vi "Update OccupancyGrid with Forget_factor.vi"(8 "error in (no error)":errorcluster, 11 "Probabilistic_OccupancyGrid in":refnum<class "Probabilistic_OccupancyGrid.lvclass">) -> (0 "error out":errorcluster, 3 "Probabilistic_OccupancyGrid out":refnum<class "Probabilistic_OccupancyGrid.lvclass">)   [LabVIEW 2017, in "Probabilistic_OccupancyGrid.lvclass"]
doc: "Update all cell costs with forget factor f\nlog(odd(ci,j.=occupied))= log(odd(ci,j.=occupied))+f *sign(log(odd(ci,j.=occupied)))\nCells not updated recently would have costs linearly reduced to 0"
uses:
  Probabilistic_OccupancyGrid.lvclass
  Probabilistic_OccupancyGrid.lvclass/Probabilistic_OccupancyGrid.ctl
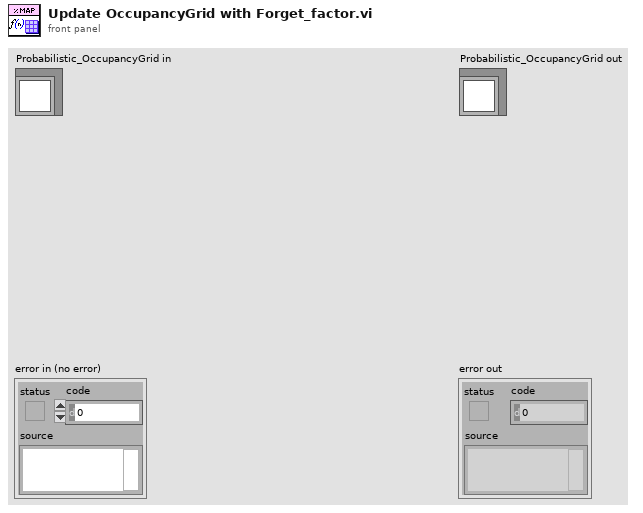
[diagram p1: front panel]
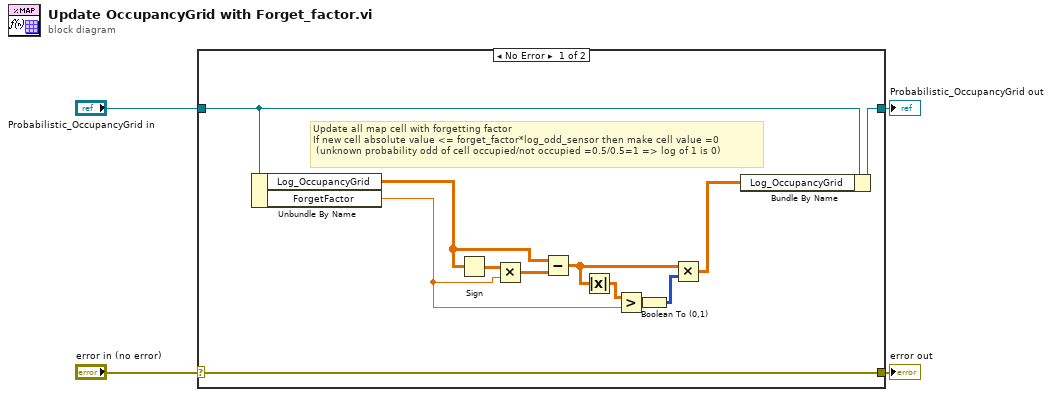
[diagram p0: block diagram]
diagram:
  n1 = case shown="No Error" "error in (no error)" {
    selector: "error in (no error)" -> [w16 w18]
    tunnel: [w16 w18] -> w3
    tunnel: [w8 w17] -> w1
    tunnel: "Probabilistic_OccupancyGrid in" -> [w9 w17]
    frame No Error {
      # "Update all map cell with forgetting factor\nIf new cell absolute value <= forget_factor*log_odd_sensor then make cell value =0\n (unknown probability odd of cell occupied/not occupied =0.5/0.5=1 => log of 1 is 0)"
      n2 = Unbundle By Name(w9) -> ("Log_OccupancyGrid"=w11:dbl[][], "ForgetFactor"=w10:dbl)
      n3 = Sign(1:w11) -> (0:w6:dbl[][])
      n4 = Multiply(x=w6, y=w10) -> (x*y=w5:dbl[][])
      n5 = Subtract(x=w11, y=w5) -> (x-y=w14:dbl[][])
      n6 = Absolute Value(x=w14) -> (abs(x)=w12:dbl[][])
      n7 = Greater?(x=w12, y=w10) -> (0:w13:bool[][])
      n8 = Boolean To (0,1)(Boolean=w13) -> (0, 1=w15:i16[][])
      n9 = Multiply(x=w14, y=w15) -> (x*y=w7:dbl[][])
      n10 = Bundle By Name(cluster=w9, "Log_OccupancyGrid"=w7) -> (w8:refnum<class "Probabilistic_OccupancyGrid.lvclass">)
    }
    frame Error {
    }
  }
  "error out" <- w3
  "Probabilistic_OccupancyGrid out" <- w1
